vi "daemon connect.vi"(8 "error in (no error)":errorcluster, 10 "port (6543)":u16=6543, 11 "address (localhost)":string="localhost") -> (0 "error out":errorcluster, 3 "daemon reference out":refnum<k5>)   [LabVIEW 2017]
doc: "<b>Description: </b> This command will connect to the Daemon software and provide a reference which can be used by the commands to interact with the Daemon session.\n\n<b>Parameters: </b> None\n____________________________________________\nDIPC 692 Daemon API 10.0.0.1\nSam Tee - Dyson Technology Ltd\nCopyright (c) 2024, Dyson Technology Ltd"
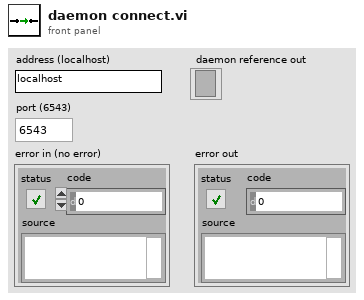
[diagram p1: front panel]
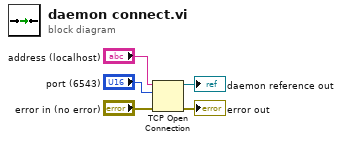
[diagram p0: block diagram]
diagram:
  n1 = TCP Open Connection(address="address (localhost)", remote port or service name="port (6543)", error in (no error)="error in (no error)") -> (connection ID=→"daemon reference out":refnum<k5>, error out=→"error out":errorcluster)  [unwired: 2 in]
